vi "getColor.vi"(8 "error in (no error)":errorcluster, 11 "junkClass01 in":refnum<class "junkClass01.lvclass">) -> (0 "error out":errorcluster, 2 "Color Box":u32, 3 "junkClass01 out":refnum<class "junkClass01.lvclass">)   [LabVIEW 2013, in "junkClass01.lvclass"]
uses:
  junkClass01.lvclass
  junkClass01.lvclass/junkClass01.ctl
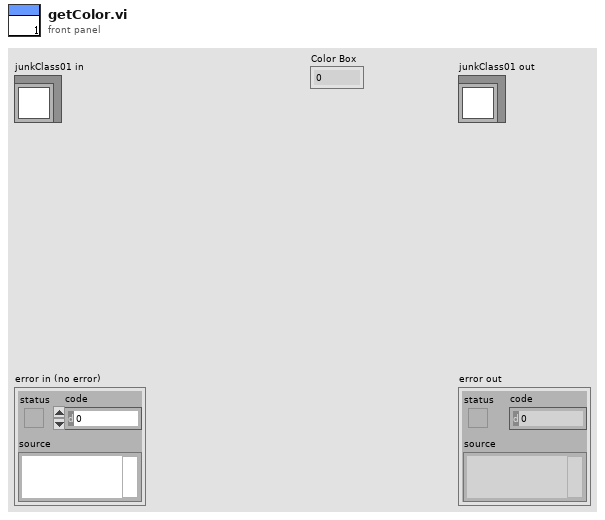
[diagram p1: front panel]
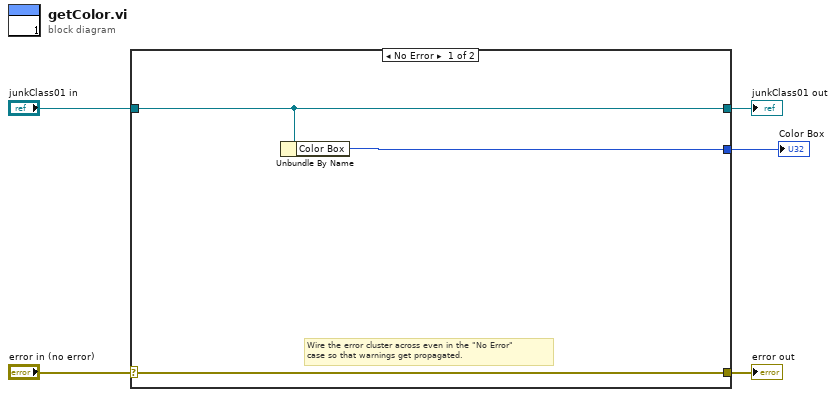
[diagram p0: block diagram]
diagram:
  n1 = case shown="No Error" "error in (no error)" {
    selector: "error in (no error)" -> [w8 w10]
    tunnel: [w8 w10] -> w4
    tunnel: [w7 w9] -> w2
    tunnel: "junkClass01 in" -> [w7 w9]
    tunnel: [w6 _] -> w1
    frame No Error {
      # "Wire the error cluster across even in the \"No Error\"\ncase so that warnings get propagated."
      n2 = Unbundle By Name(w7) -> ("Color Box"=w6:u32)
    }
    frame Error {
    }
  }
  "error out" <- w4
  "junkClass01 out" <- w2
  "Color Box" <- w1
